vi "UserLeverCheck.vi"(7 "Enum":T1, 8 "error in (no error)":errorcluster, 10 "User Name":string) -> (0 "error IO":errorcluster, 1 "User Level":string)   [LabVIEW 2021]
uses:
  UserLevel.ctl
  <vilib>/Utility/file.llb/Read Delimited Spreadsheet (string).vi
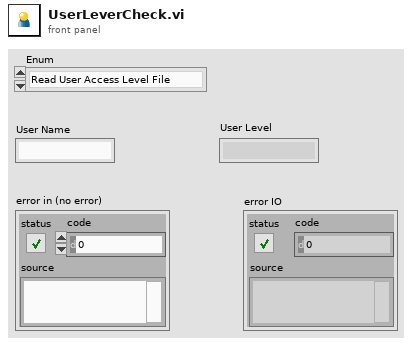
[diagram p1: front panel]
types:
  T1 = typedef "UserLevel.ctl" = enum16{"Read User Access Level File", "Set Current User", "Get User Access Level"}
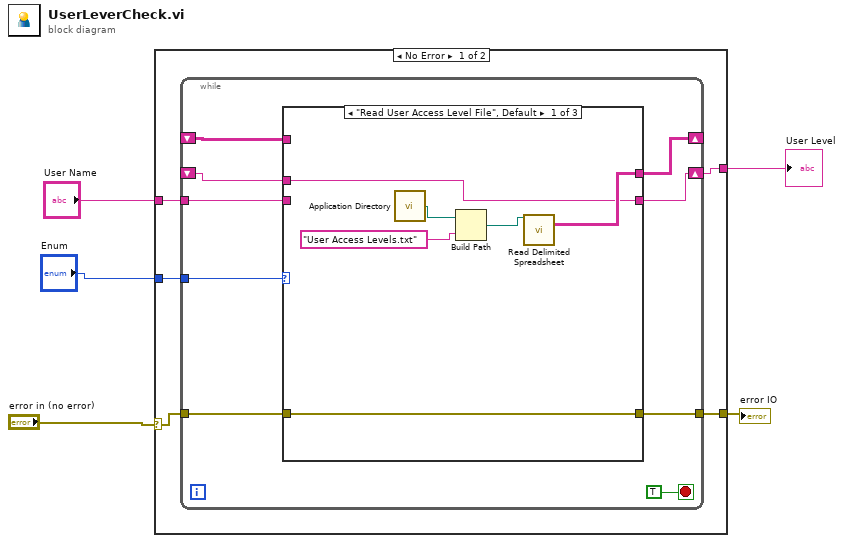
[diagram p0: block diagram]
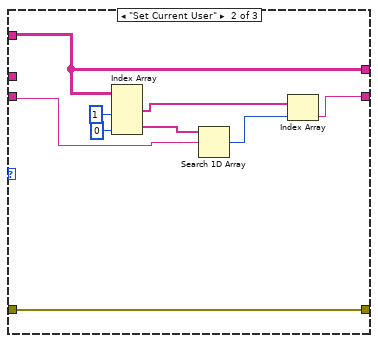
[diagram p2: hidden frame]
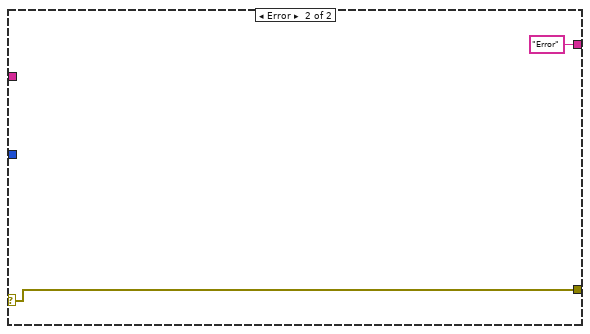
[diagram p4: hidden frame]
diagram:
  n1 = case shown="No Error" "error in (no error)" {
    selector: "error in (no error)" -> [w7 w39]
    tunnel: "Enum" -> [w10 _]
    tunnel: "User Name" -> [w9 _]
    tunnel: [w8 w39] -> w2
    tunnel: [w6 "Error" ("String")] -> w1
    frame No Error {
      n2 = while {
        tunnel: w10 -> [w18]
        tunnel: w9 -> [w17]
        shift-right: [w16] -> _
        shift-left: _ -> [w15]
        shift-right: [w14] -> w6
        shift-left: _ -> [w13]
        tunnel: [w12] -> w8
        tunnel: w7 -> [w11]
        stop <- TRUE stop-if-true
        n3 = case shown="\"Read User Access Level File\", Default" w18 {
          tunnel: w17 -> [_ w31 _]
          tunnel: [w22 w27 w37] -> w16
          tunnel: w15 -> [_ w27 w37]
          tunnel: [w21 w28 w36] -> w14
          tunnel: w13 -> [w21 _ w36]
          tunnel: [w20 w26 w35] -> w12
          tunnel: w11 -> [w20 w26 w35]
          frame "Read User Access Level File", Default {
            n4 = call <vilib>:"Application Directory.vi"() -> ("Application Directory"=w25:path)
            n5 = Build Path(base path=w25, name or relative path="User Access Levels.txt") -> (appended path=w23:path)
            n6 = call-poly <vilib>:"Read Delimited Spreadsheet.vi"("file path (dialog if empty)"=w23) -> ("all rows"=w22:string[][])  [unwired: 9 in, 5 out]
          }
          frame "Set Current User" {
            n7 = Index Array(array=w27, index (col) #1=1 ("disabled index (col)"), index (col) #2=0 ("index (col)")) -> (element #1=w30:string[], element #2=w32:string[])  [unwired: 2 in]
            n8 = Search 1D Array(1D array=w32, element=w31) -> (index of element=w29:i32)  [unwired: 1 in]
            n9 = Index Array(array=w30, index=w29) -> (element=w28:string)
          }
          frame "Get User Access Level" {
          }
        }
      }
    }
    frame Error {
    }
  }
  "error IO" <- w2
  "User Level" <- w1
